vi "SetValueByArrayIndex.vi"(0 "VI Reference In":refnum<vi>, 2 "delimiter (>>)":string=">>", 5 "Control Path":string, 7 "Index Array":i32[](array[numeric]), 11 "Error In":errorcluster) -> (4 "VI Reference Out":refnum<vi>, 15 "Error Out":errorcluster)   [LabVIEW 2016, in "Drona.lvlib" / "ControlValue.lvlib" / "StimulusListbox.lvlib"]
doc: "Sets value(signaling) for the multi select listbox control whose index values are specified. \n\nThe input control name is given as a string , incase of path, use delimiters inbetween the path."
uses:
  StimulusListbox.lvlib
  <vilib>/Utility/error.llb/Error Cluster From Error Code.vi
  <vilib>/ErrorRing/Error Ring.xnode
  Drona.lvlib
  Get/GetControlRef/GetControlRef.lvlib
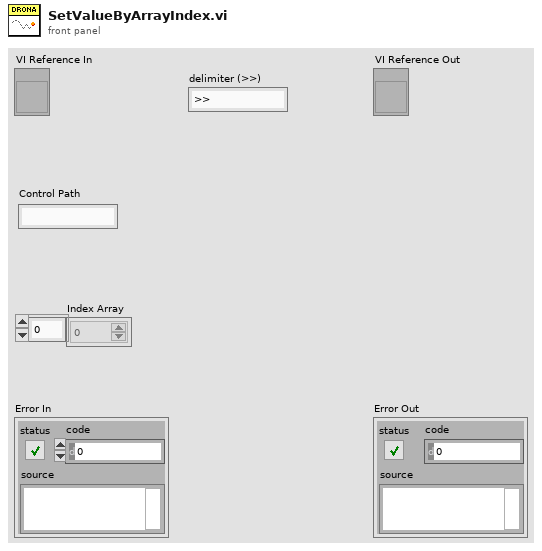
[diagram p1: front panel]
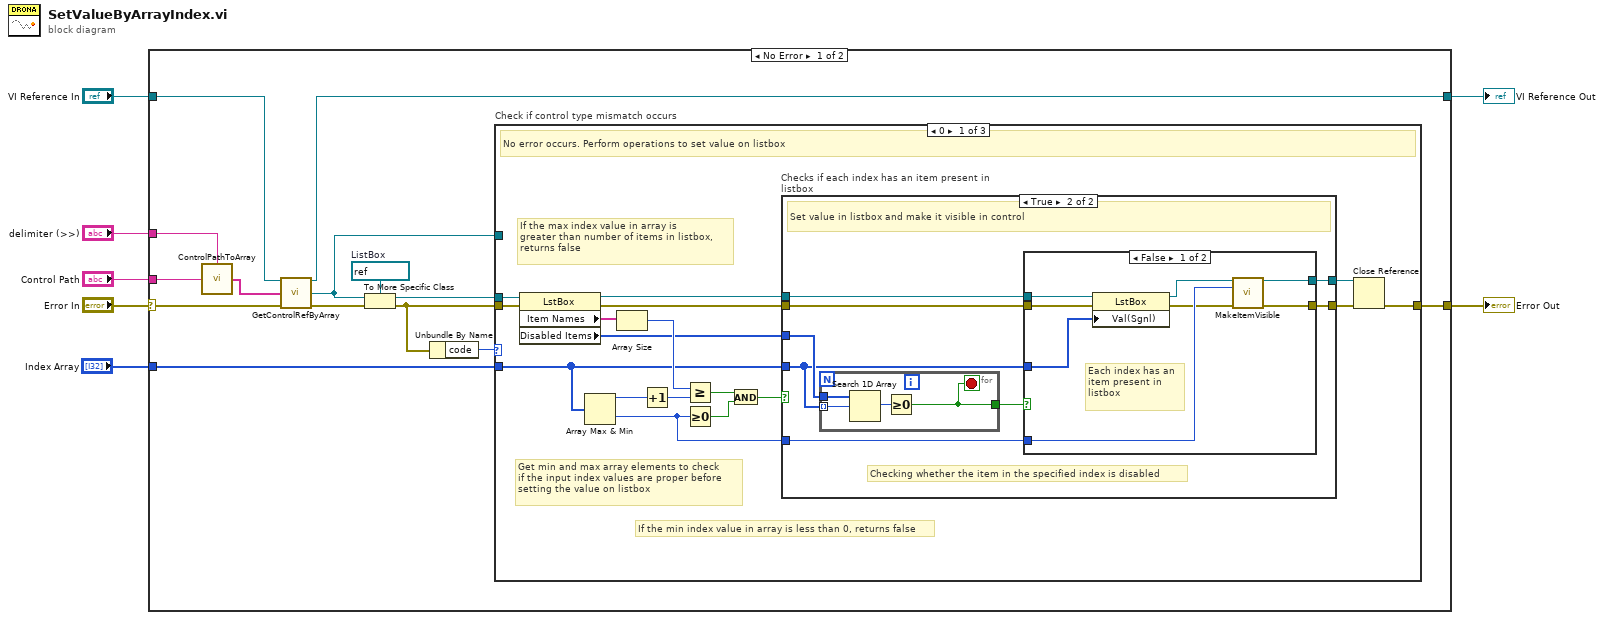
[diagram p0: block diagram]
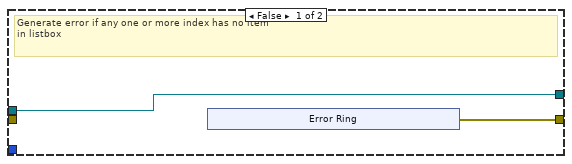
[diagram p2: hidden frame]
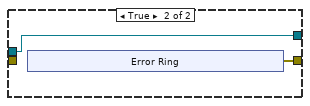
[diagram p3: hidden frame]
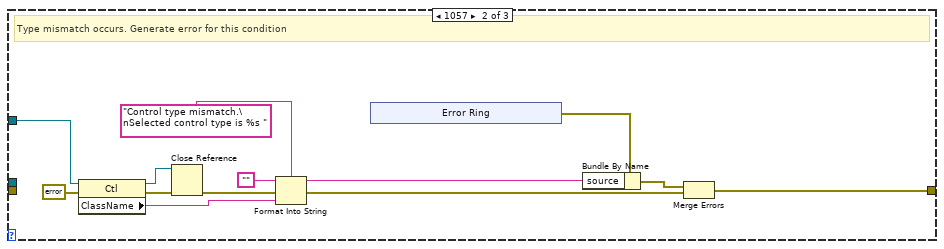
[diagram p4: hidden frame]
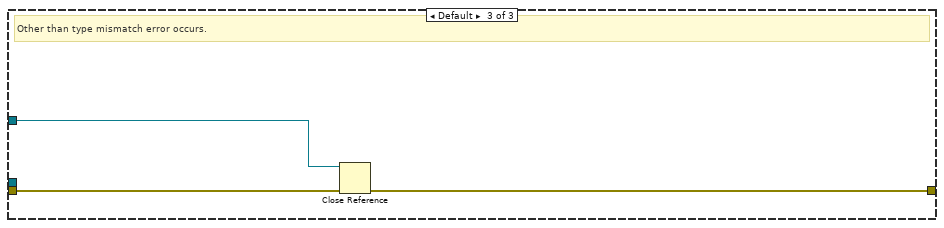
[diagram p5: hidden frame]
diagram:
  n1 = case shown="No Error" "Error In" {
    selector: "Error In" -> [w16 w95]
    tunnel: [w17 w95] -> w6
    tunnel: "VI Reference In" -> [w14 w94]
    tunnel: "Control Path" -> [w20 _]
    tunnel: "Index Array" -> [w11 _]
    tunnel: [w13 w94] -> w2
    tunnel: "delimiter (>>)" -> [w19 _]
    frame No Error {
      w21 = refnum<vi> refnum  # ListBox
      n2 = call "ControlPathToArray.vi"("Control Name"=w20, "delimiter (>>)"=w19) -> ("Control Path"=w15:string[])
      n3 = call "GetControlRefByArray.vi"("VI Reference In"=w14, "Control Path"=w15, "error In"=w16) -> ("VI Reference Out"=w13:refnum<vi>, "Ctl Refnum"=w8:refnum<vi>, "error out"=w12:errorcluster)  [unwired: 10 in]
      n4 = To More Specific Class(target class=w21, reference=w8, error in=w12) -> (specific class reference=w18:refnum<vi>, error out=w10:errorcluster)
      n5 = Unbundle By Name(w10) -> ("code"=w9:i32)
      n6 = case "Check if control type mismatch occurs" shown="0" w9 {
        tunnel: w10 -> [w38 _ w93]
        tunnel: w18 -> [w34 _ _]
        tunnel: [w29 w73 w92] -> w17
        tunnel: w11 -> [w24 _ _]
        tunnel: w8 -> [_ w74 w91]
        frame 0 {
          # "If the min index value in array is less than 0, returns false"
          # "If the max index value in array is \ngreater than number of items in listbox, \nreturns false"
          # "Get min and max array elements to check \nif the input index values are proper before \nsetting the value on listbox"
          # "No error occurs. Perform operations to set value on listbox"
          n7 = property class="LstBox"(reference=w34, error in=w38) -> (reference out=w33:refnum<vi>, error out=w35:errorcluster, "Item Names"=w32:string[], "Disabled Items"=w22:i32[])
          n8 = Array Max & Min(array=w24) -> (max value=w28:i32, min value=w26:i32)  [unwired: 2 out]
          n9 = Array Size(array=w32) -> (size(s)=w31:i32)
          n10 = Increment(x=w28) -> (x+1=w27:i32)
          n11 = Greater Or Equal?(x=w31, y=w27) -> (x >= y?=w25:bool)
          n12 = Greater Or Equal To 0?(x=w26) -> (x >= 0?=w23:bool)
          n13 = And(x=w25, y=w23) -> (x .and. y?=w30:bool)
          n14 = case "Checks if each index has an item present in listbox" shown="True" w30 {
            tunnel: [w39 w53] -> w37
            tunnel: [w40 w52] -> w36
            tunnel: w26 -> [_ w51]
            tunnel: w35 -> [_ w50]
            tunnel: w33 -> [w40 w49]
            tunnel: w24 -> [_ w47]
            tunnel: w22 -> [_ w48]
            frame False {
              # "Generate error if any one or more index has no item \nin listbox"
              n15 = xnode "Error Ring"() -> ("error out"=w39:errorcluster)
            }
            frame True {
              # "Checking whether the item in the specified index is disabled"
              # "Set value in listbox and make it visible in control"
              n16 = for {
                tunnel: w47 -> [w56] mode=indexing
                tunnel: w48 -> [w57]
                tunnel: [w54] -> w46
                stop <- w54 stop-if-true
                n17 = Search 1D Array(1D array=w57, element=w56) -> (index of element=w55:i32)  [unwired: 1 in]
                n18 = Greater Or Equal To 0?(x=w55) -> (x >= 0?=w54:bool)
              }
              n19 = case shown="False" w46 {
                tunnel: [w65 w66] -> w53
                tunnel: [w64 w67] -> w52
                tunnel: w51 -> [w63 _]
                tunnel: w50 -> [w62 _]
                tunnel: w49 -> [w60 w67]
                tunnel: w47 -> [w59 _]
                frame False {
                  # "Each index has an item present in listbox"
                  n20 = property class="LstBox"(reference=w60, error in=w62, "Val(Sgnl)"=w59) -> (reference out=w58:refnum<vi>, error out=w61:errorcluster)
                  n21 = call "MakeItemVisible.vi"("ListBox Ref In"=w58, "Item Index"=w63, "Error In"=w61) -> ("ListBox Ref Out"=w64:refnum<vi>, "Error Out"=w65:errorcluster)  [unwired: 11 in]
                }
                frame True {
                  n22 = xnode "Error Ring"() -> ("error out"=w66:errorcluster)
                }
              }
            }
          }
          n23 = Close Reference(reference=w36, error in (no error)=w37) -> (error out=w29:errorcluster)
        }
        frame 1057 {
          # "Type mismatch occurs. Generate error for this condition"
          n24 = property class="Ctl"(reference=w74, error in=errorcluster {"status"=FALSE, "code"=0, "source"=""} ("error out")) -> (reference out=w75:refnum<vi>, error out=w85:errorcluster, "ClassName"=w82:string)
          n25 = Close Reference(reference=w75, error in (no error)=w85) -> (error out=w76:errorcluster)
          n26 = Format Into String(format string="Control type mismatch.\nSelected control type is %s ", initial string="", error in=w76, w82) -> (resulting string=w79:string, error out=w77:errorcluster)
          n27 = xnode "Error Ring"() -> ("error out"=w80:errorcluster)
          n28 = Bundle By Name(cluster=w80, "source"=w79) -> (w78:errorcluster)
          n29 = Merge Errors(w78, w77) -> (w73:errorcluster)
        }
        frame Default {
          # "Other than type mismatch error occurs."
          n30 = Close Reference(reference=w91, error in (no error)=w93) -> (error out=w92:errorcluster)
        }
      }
    }
    frame Error {
    }
  }
  "Error Out" <- w6
  "VI Reference Out" <- w2
